vi "Page_Source_Settings_CustVISettings_UpdateDisplay.vi"(8 "error in (no error)":errorcluster, 9 "sourceInclusion":T1, 10 "sourceProperties in":T2[](array[typedef]), 11 "AB_EXE in":refnum<class "AB_EXE.lvclass">) -> (0 "error out":errorcluster, 1 "Run when opened disabled state":u8, 2 "sourceProperties out":T2[](array[typedef]), 3 "AB_EXE out":refnum<class "AB_EXE.lvclass">, 5 "AEH disabled state":u8)   [LabVIEW 2020, in "AB_EXE.lvclass"]
uses:
  <vilib>/AppBuilder/AB_Classes/EXE/AB_EXE.lvclass
  <vilib>/AppBuilder/AB_Classes/EXE/AB_EXE.lvclass/AB_EXE.ctl
  <vilib>/AppBuilder/AB_Source_Property_Type.ctl
  <vilib>/AppBuilder/AB_Classes/Application/AB_Application.lvclass
  <vilib>/AppBuilder/AB_Source_Properties.ctl
  <vilib>/AppBuilder/AB_Source_Inclusion.ctl
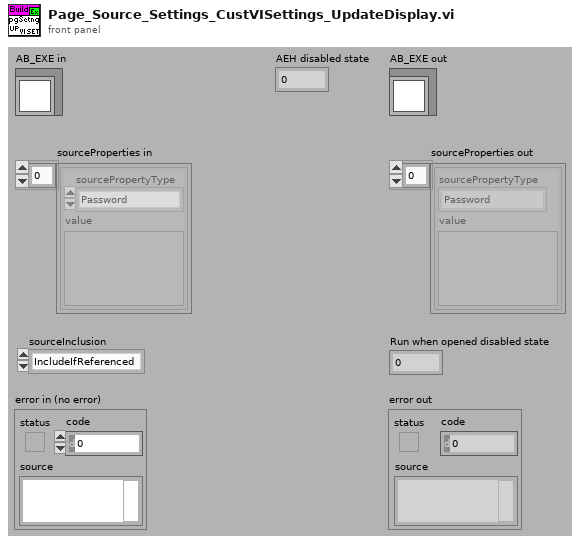
[diagram p1: front panel]
types:
  T1 = typedef "AB_Source_Inclusion.ctl" = enum16{"IncludeIfReferenced", "Include", "Exclude", "TopLevel"}
  T2 = typedef "AB_Source_Properties.ctl" = cluster{"sourcePropertyType":T3, "value":variant}
  T3 = typedef "AB_Source_Property_Type.ctl" = enum16{"Remove block diagram", "Remove front panel", "Password", "Window has title bar", "Show menu bar", "Show vertical scroll bar", "Show horizontal scroll bar", "Show toolbar", "Show Abort button", "Show fp when called", "Window behavior", "Allow user to close window", "Window run-time position", "Run when opened", "Allow debugging", "Auto error handling", "Generate guard code", "Use stack variables", "Expression folding", "Integer only", "Inline subVI"}
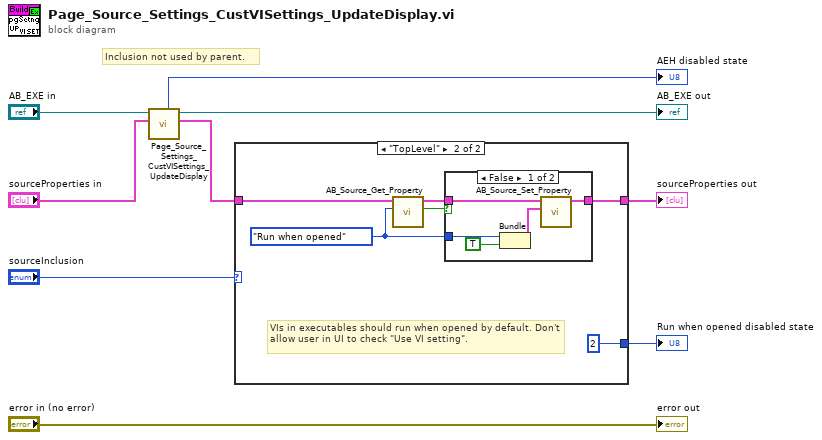
[diagram p0: block diagram]
diagram:
  # "Inclusion not used by parent."
  n1 = call-parent "Page_Source_Settings_CustVISettings_UpdateDisplay.vi"("sourceProperties in"="sourceProperties in", "AB_Application in"="AB_EXE in") -> ("sourceProperties out"=w1:T2[], "AB_Application out"=→"AB_EXE out":refnum<class "AB_EXE.lvclass">, "AEH disabled state"=→"AEH disabled state":u8)  [unwired: 5 in, 2 out]
  n2 = case shown="\"TopLevel\"" "sourceInclusion" {
    tunnel: w1 -> [w10 w16]
    tunnel: [w10 w15] -> w8
    tunnel: [_ u8 2 ("Run when opened disabled state")] -> w7
    frame Default {
    }
    frame "TopLevel" {
      w11 = AB_Source_Property_Type."Run when opened" ("type")
      # "VIs in executables should run when opened by default. Don't allow user in UI to check \"Use VI setting\"."
      n3 = call <vilib>:"AB_Source_Get_Property.vi"("type"=w11, "sourceProperties in"=w16) -> ("found"=w12:bool, "sourceProperties out"=w13:T2[])  [unwired: 6 in, 2 out]
      n4 = case shown="False" w12 {
        tunnel: w13 -> [w21 w22]
        tunnel: [w20 w22] -> w15
        tunnel: w11 -> [w19 _]
        frame False {
          n5 = Bundle("type"=w19, TRUE) -> (w17:cluster{"type":T3, bool})  [unwired: 1 in]
          n6 = call <vilib>:"AB_Source_Set_Property.vi"("sourceProperty"=w17, "sourceProperties in"=w21) -> ("sourceProperties out"=w20:T2[])  [unwired: 7 in, 2 out]
        }
        frame True {
        }
      }
    }
  }
  "sourceProperties out" <- w8
  "Run when opened disabled state" <- w7
  "error out" <- "error in (no error)"
